vi "Write Function Parameters.vi"(0 "signal configuration":refnum<class "SV Function.lvclass">, 1 "function type":u16(ring) items=["Sine", "Triangle", "Square", "Sawtooth"], 5 "frequency (Hz)":dbl=1000.0, 7 "amplitude":dbl=1.0, 9 "phase (deg)":dbl, 11 "error in (no error)":errorcluster) -> (4 "signal configuration":refnum<class "SV Function.lvclass">, 15 "error out":errorcluster)   [LabVIEW 2017, in "SV Function.lvclass"]
uses:
  <vilib>/addons/_NISVFA/_Generation/Signal Generation/SV Function/SV Function.lvclass
  <vilib>/addons/_NISVFA/_Generation/Signal Generation/SV Function/SV Function.lvclass/SV Function.ctl
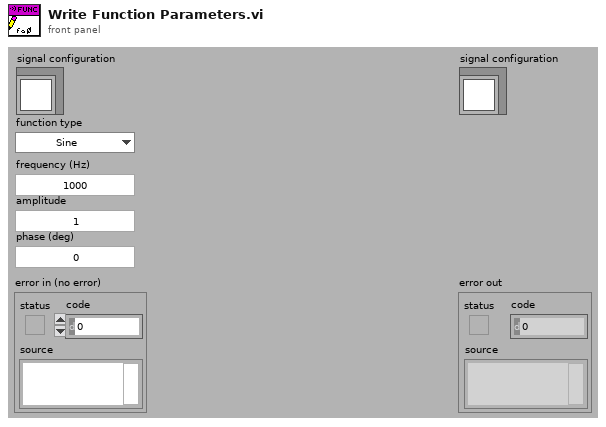
[diagram p1: front panel]
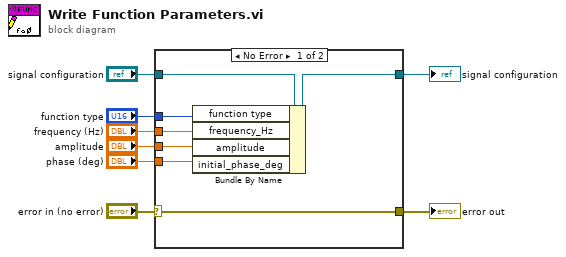
[diagram p0: block diagram]
diagram:
  n1 = case shown="No Error" "error in (no error)" {
    selector: "error in (no error)" -> [w10 w16]
    tunnel: [w10 w16] -> w7
    tunnel: [w9 w17] -> w2
    tunnel: "signal configuration" -> [w15 w17]
    tunnel: "frequency (Hz)" -> [w11 _]
    tunnel: "amplitude" -> [w14 _]
    tunnel: "phase (deg)" -> [w13 _]
    tunnel: "function type" -> [w12 _]
    frame No Error {
      n2 = Bundle By Name(cluster=w15, "function type"=w12, "frequency_Hz"=w11, "amplitude"=w14, "initial_phase_deg"=w13) -> (w9:refnum<class "SV Function.lvclass">)
    }
    frame Error {
    }
  }
  "error out" <- w7
  "signal configuration" <- w2
